vi "Cache Destination State.vi"(0 "TLB' Template in":refnum<class "TLB` - {TMPL}.lvclass">, 5 "state in":string) -> (4 "TLB' Template out":refnum<class "TLB` - {TMPL}.lvclass">)   [LabVIEW 2015, in "TLB` Template.lvlib" / "TLB` - {TMPL}.lvclass"]
uses:
  TLB` - {TMPL}.lvclass
  TLB` - {TMPL}.lvclass/TLB` - {TMPL}.ctl
  Error Handler/TLB` Error Handler.lvclass/TLB` Error Handler.ctl
  Error Handler/accessors/Set Destination State.vi
  Error Handler/TLB` Error Handler.lvclass
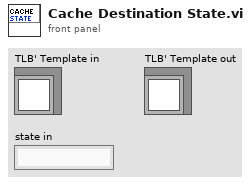
[diagram p1: front panel]
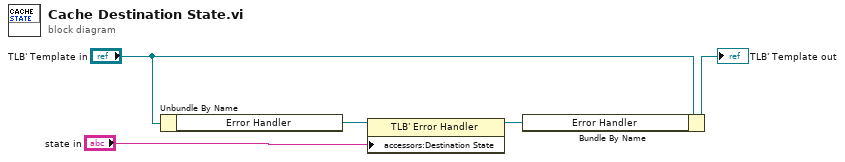
[diagram p0: block diagram]
diagram:
  n1 = Unbundle By Name("TLB' Template in") -> ("Error Handler"=w3:refnum<class "TLB` Error Handler.lvclass">)
  n2 = property class="TLB' Error Handler"(reference=w3, "accessors:Destination State"="state in") -> (reference out=w2:refnum<class "TLB` Error Handler.lvclass">)  [unwired: 1 in, 1 out]
  n3 = Bundle By Name(cluster="TLB' Template in", "Error Handler"=w2) -> (→"TLB' Template out":refnum<class "TLB` - {TMPL}.lvclass">)
